vi "PQntuples.vi"(8 "error in (no error)":errorcluster, 10 "res":u64) -> (0 "error out":errorcluster, 1 "PQnTuples":i64, 2 "res out":u64)   [LabVIEW 2019, in "libpqlv64.lvlib"]
doc: "Returns the number of rows (tuples) in the query result."
uses:
  libpqlv64.lvlib
  libpq.dll
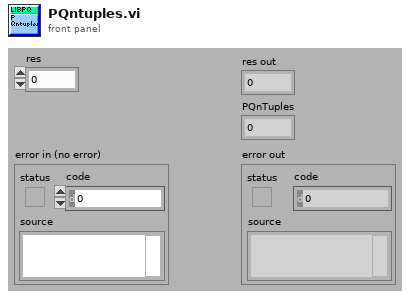
[diagram p1: front panel]
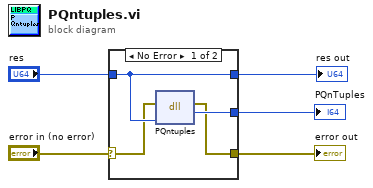
[diagram p0: block diagram]
diagram:
  n1 = case shown="No Error" "error in (no error)" {
    selector: "error in (no error)" -> [w7 w11]
    tunnel: [w6 w11] -> w4
    tunnel: "res" -> [w8 w10]
    tunnel: [w9 _] -> w2
    tunnel: [w8 w10] -> w1
    frame No Error {
      n2 = dll-call lib="libpq.*" fn="PQntuples"(error in=w7, "res"=w8) -> (error out=w6:errorcluster, "PQnTuples"=w9:i64)  [unwired: 3 in, 1 out]
    }
    frame Error {
    }
  }
  "PQnTuples" <- w2
  "error out" <- w4
  "res out" <- w1
